vi "VariantToString.vi"(10 "error in (no error)":errorcluster, 11 "Variant":variant) -> (2 "error out":errorcluster, 3 "Value":string)   [LabVIEW 2019, in "Utilities.lvlib"]
uses:
  Utilities.lvlib
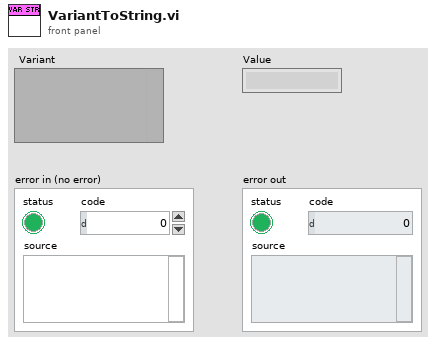
[diagram p1: front panel]
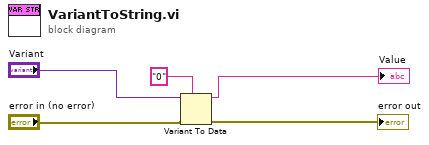
[diagram p0: block diagram]
diagram:
  n1 = Variant To Data(error in="error in (no error)", type="0", Variant="Variant") -> (data=→"Value":string, error out=→"error out":errorcluster)
